vi "RP read file.vi"(8 "Error In":errorcluster) -> (0 "Error Out":errorcluster)   [LabVIEW 2015]
uses:
  <vilib>/Waveform/WDTOps.llb/WDT Number of Waveform Samples DBL.vi
  <vilib>/measure/NI_MABase.lvlib
panel:
  in  "offset":dbl format="%0.2p"
  in  "amplitude":dbl=1.0 format="%0.2p"
  in  "Pipeline delay":dbl=-247.0
  out "Frequency":dbl format="%_19p"
  out "Phase":u32
  out "Frequency word":u32
  out "Waveform Graph":waveform(dbl)[](graph)
  out "group/channel names":string[][](array[string])
  in  "File Path Control":path
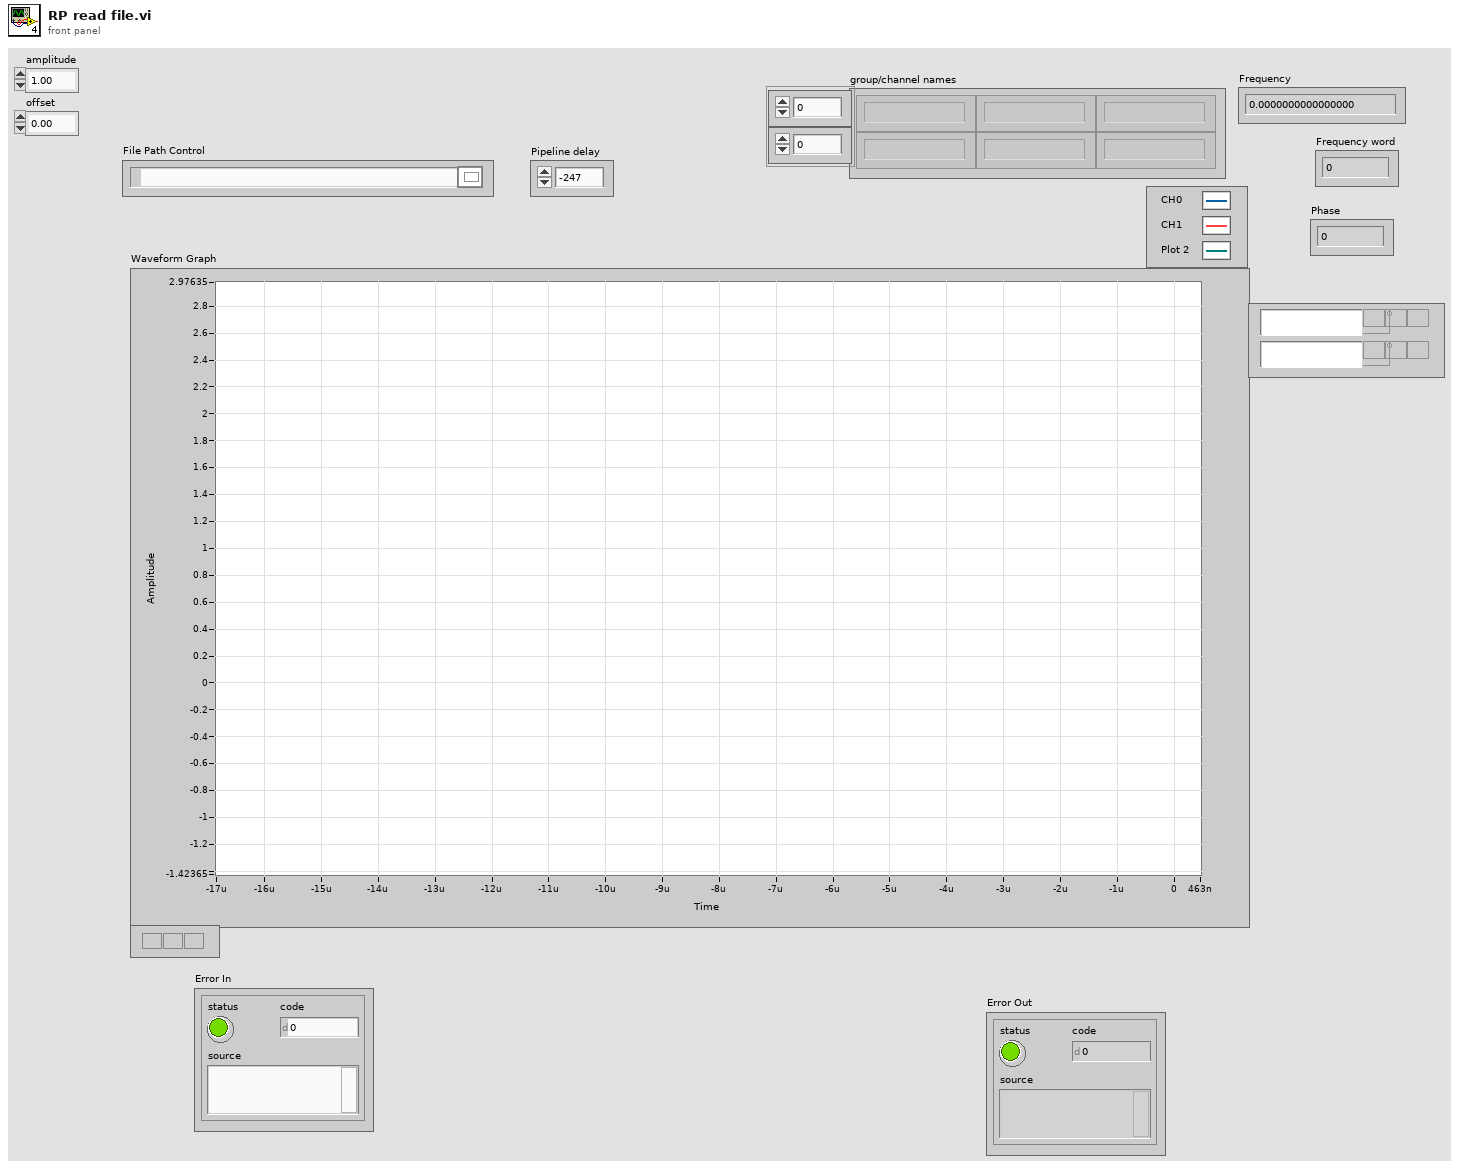
[diagram p1: front panel]
types:
  T1 = enum16{"open", "open or create", "create or replace", "create", "open (read-only)"}
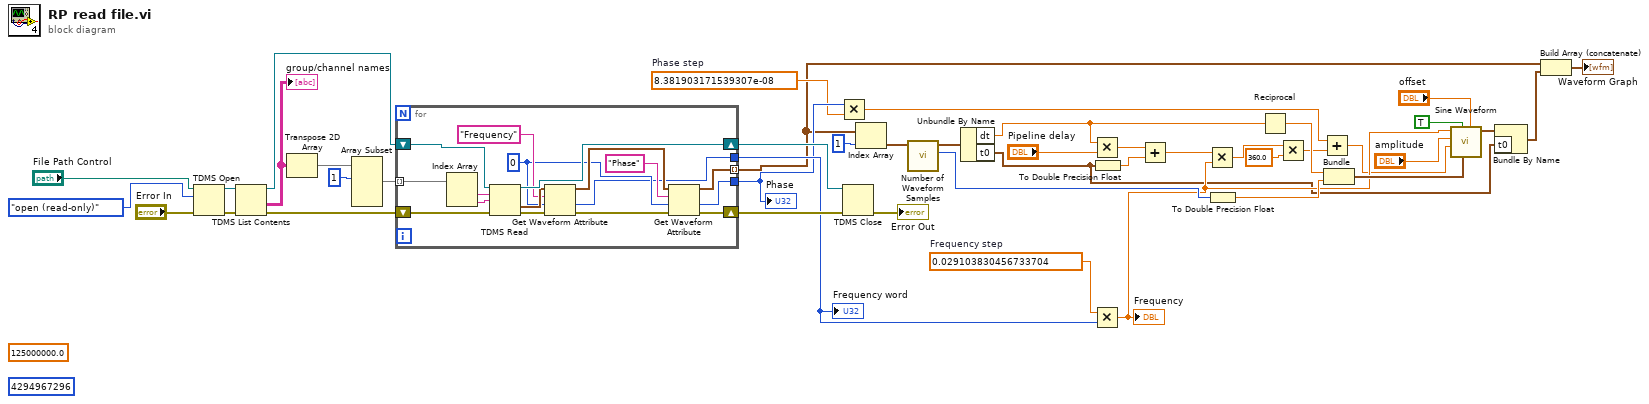
[diagram p0: block diagram]
diagram:
  w24 = 8.381903171539307e-08  # Phase step
  w27 = 0.029103830456733704  # Frequency step
  (unwired) u64 4294967296
  (unwired) 125000000.0
  n1 = TDMS Open(8:"Error In", 10:T1."open (read-only)" ("operation (0:open)"), 11:"File Path Control") -> (0:w41:errorcluster, 3:w40:refnum<k34>)  [unwired: 4 in]
  n2 = TDMS List Contents(4:w41, 7:w40) -> (0:w39:errorcluster, 1:w37:string[][], 3:w38:refnum<k34>)  [unwired: 1 in, 1 out]
  "group/channel names" <- w37
  n3 = Transpose 2D Array(2D array=w37) -> (transposed array=w32:string[][])
  n4 = Array Subset(array=w32, index (row)=1 ("index")) -> (w33:string[][])  [unwired: 3 in]
  n5 = for {
    shift-right: [w49] -> w35
    shift-left: w39 -> [w61]
    shift-right: [w56] -> w36
    shift-left: w38 -> [w60]
    tunnel: w33 -> [w59] mode=indexing
    tunnel: [w51] -> w9 mode=indexing
    tunnel: [w46] -> w26
    tunnel: [w45] -> w25
    w47 = u32 0 ("index")
    n6 = Index Array(array=w59) -> (element #1=w57:string, element #2=w58:string)  [unwired: 2 in]
    n7 = TDMS Read(0:w60, 5:w57, 7:w58, 11:w61) -> (4:w56:refnum<k34>, 10:w55:waveform(dbl), 15:w53:errorcluster)  [unwired: 4 in, 3 out]
    n8 = Get Waveform Attribute(4:w53, 5:w47, 6:"Frequency" ("name"), 7:w55) -> (0:w50:errorcluster, 1:w46:u32, 3:w52:waveform(dbl))  [unwired: 1 out]
    n9 = Get Waveform Attribute(4:w50, 5:w47, 6:"Phase" ("name"), 7:w52) -> (0:w49:errorcluster, 1:w45:u32, 3:w51:waveform(dbl))  [unwired: 1 out]
  }
  "Frequency word" <- w26
  "Phase" <- w25
  n10 = Multiply(x=w25, y=w24) -> (x*y=w14:dbl)
  n11 = TDMS Close(8:w35, 11:w36) -> (0:→"Error Out":errorcluster)  [unwired: 1 out]
  n12 = Index Array(array=w9, index=1) -> (element=w29:waveform(dbl))
  n13 = call-poly <vilib>:"Number of Waveform Samples.vi"("waveform in"=w29) -> ("number of samples"=w23:i32, "waveform out"=w28:waveform(dbl))  [unwired: 8 in, 1 out]
  n14 = Unbundle By Name(w28) -> ("dt"=w5:dbl, "t0"=w10:timestamp)
  n15 = Multiply(x=w5, y="Pipeline delay") -> (x*y=w3:dbl)
  n16 = Multiply(x=w27, y=w26) -> (x*y=w18:dbl)
  "Frequency" <- w18
  n17 = To Double Precision Float(number=w10) -> (double precision float=w17:dbl)
  n18 = Add(x=w3, y=w17) -> (x+y=w4:dbl)
  n19 = Multiply(x=w4, y=w18) -> (x*y=w16:dbl)
  n20 = To Double Precision Float(number=w23) -> (double precision float=w21:dbl)
  n21 = Reciprocal(x=w5) -> (1/x=w22:dbl)
  n22 = Multiply(x=w16, y=360.0) -> (x*y=w13:dbl)
  n23 = Add(x=w14, y=w13) -> (x+y=w12:dbl)
  n24 = Bundle(w22, w21) -> (w20:cluster{dbl, dbl})  [unwired: 1 in]
  n25 = call <vilib>:"Sine Waveform.vi"("offset"="offset", "sampling info"=w20, "reset signal"=TRUE, "phase"=w12, "amplitude"="amplitude", "frequency"=w18) -> ("signal out"=w11:waveform(dbl))  [unwired: 4 in, 1 out]
  n26 = Bundle By Name(cluster=w11, "t0"=w10) -> (w8:waveform(dbl))
  n27 = Build Array (concatenate)(w9, w8) -> (→"Waveform Graph":waveform(dbl)[])
